vi "Do Event Report.vi"(8 "error in (no error)":errorcluster, 9 "Event Data":variant, 10 "Report Events":T1=enum."Inited", 11 "Caller Enqueuer":refnum<class "Message Enqueuer.lvclass">) -> (0 "error out":errorcluster, 3 "Message Enqueuer out":refnum<class "Message Enqueuer.lvclass">)   [LabVIEW 2020, in "Actor_AFG.lvlib" / "Actor_AFG.lvclass"]
uses:
  Actor_AFG.lvclass
  <vilib>/ActorFramework/Message Enqueuer/Message Enqueuer.lvclass
  AFG_Event.ctl
  I_AFG Messages/AFG Report Event Msg/AFG Report Event Msg.lvclass/AFG Report Event Msg.ctl
  <vilib>/ActorFramework/Message Enqueuer/Message Enqueuer.lvclass/Message Enqueuer.ctl
  <vilib>/ActorFramework/Message Enqueuer/Enqueue.vi
  I_AFG Messages/AFG Report Event Msg/AFG Report Event Msg.lvclass
  C:/Program Files/National Instruments/LabVIEW 2020/vi.lib/ActorFramework/Message/Message.lvclass
  <vilib>/ActorFramework/Message Priority Queue/Priority Enqueue.vi
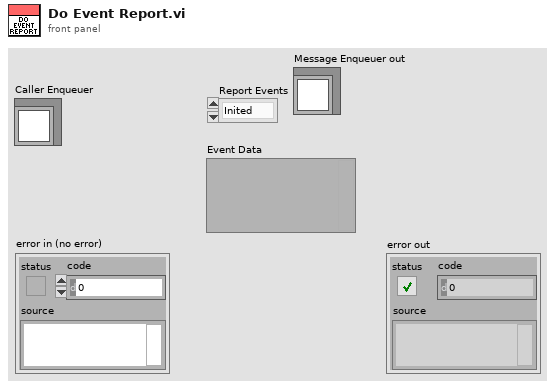
[diagram p1: front panel]
types:
  T1 = typedef "Actor_AFG.lvlib/Actor_AFG.lvclass/AFG_Event.ctl" = enum16{"General Event", "Inited", "Output", "Waveform Set", "Error"}
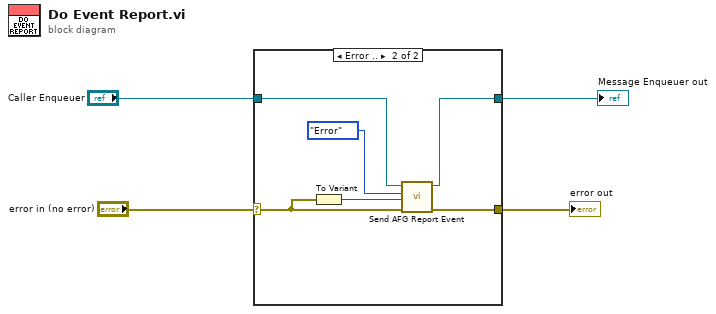
[diagram p0: block diagram]
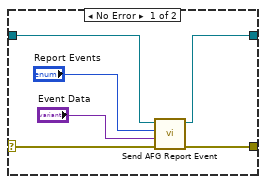
[diagram p2: hidden frame]
diagram:
  n1 = case shown="Error .." "error in (no error)" {
    selector: "error in (no error)" -> [w6 w13]
    tunnel: "Caller Enqueuer" -> [w10 w15]
    tunnel: [w7 w14] -> w2
    tunnel: [w5 w11] -> w1
    frame No Error {
      n2 = call "Send AFG Report Event.vi"("error in (no error)"=w6, "Event Data"="Event Data", "Report Events"="Report Events", "Message Enqueuer"=w10) -> ("error out"=w7:errorcluster, "Message Enqueuer out"=w5:refnum<class "Message Enqueuer.lvclass">)  [unwired: 6 in]
    }
    frame Error {
      n3 = To Variant(anything=w13) -> (Variant=w12:variant)
      n4 = call "Send AFG Report Event.vi"("error in (no error)"=w13, "Event Data"=w12, "Report Events"=AFG_Event."Error" ("Report Events 2"), "Message Enqueuer"=w15) -> ("error out"=w14:errorcluster, "Message Enqueuer out"=w11:refnum<class "Message Enqueuer.lvclass">)  [unwired: 6 in]
    }
  }
  "error out" <- w2
  "Message Enqueuer out" <- w1
